vi "FaultSetValue.vi"(9 "FaultValueToSet":dbl, 10 "Channel":string) -> (0 "error out":errorcluster, 1 "FaultValueToSet out":dbl, 2 "Channel out":string)   [LabVIEW 2015, in "MiscHelperVIs.lvlib"]
uses:
  MiscHelperVIs.lvlib
  <vilib>/NI Veristand/Execution/ChannelFaultManager/NI_VS ChannelFault ExecutionAPI.lvlib
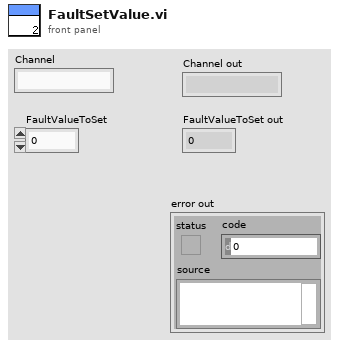
[diagram p1: front panel]
types:
  T1 = typedef "MiscHelperVIs.lvlib/VeriStand dotNet References.ctl" = cluster{"Project Ref":refnum<k24>, "Workspace Manager Ref":refnum<k24>, "Model Manager Ref":refnum<k24>, "Channel Fault Manager Ref":refnum<k24>}
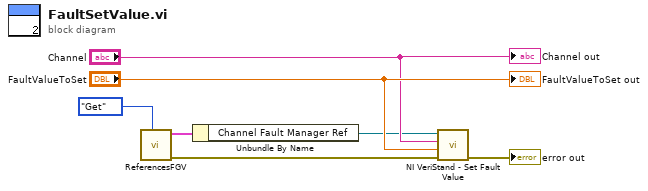
[diagram p0: block diagram]
diagram:
  n1 = call "ReferencesFGV.vi"("Get/Set"=enum16{"Get", "Set"}."Get") -> ("error out"=w1:errorcluster, "VeriStand dotNET Refs out"=w4:T1)  [unwired: 9 in]
  n2 = Unbundle By Name(w4) -> ("Channel Fault Manager Ref"=w2:refnum<k24>)
  n3 = call <vilib>:"NI VeriStand - Set Fault Value.vi"("error in (no error)"=w1, "Fault Value"="FaultValueToSet", "Channel"="Channel", "ChannelFault in"=w2) -> ("error out"=→"error out":errorcluster)  [unwired: 6 in, 1 out]
  "Channel out" <- "Channel"
  "FaultValueToSet out" <- "FaultValueToSet"
